vi "Generate Tree Data Representation.vi"(8 "error in (no error)":errorcluster, 11 "ParseGDSII in":refnum<class "ParseGDSII.lvclass">) -> (0 "error out":errorcluster, 3 "ParseGDSII out":refnum<class "ParseGDSII.lvclass">)   [LabVIEW 2019, in "ParseGDSII.lvclass"]
uses:
  ParseGDSII.lvclass
  Tree/Tree.lvclass
  ParseGDSII.lvclass/ParseGDSII.ctl
  Fast Tree/Fast Tree.lvclass
  DataTypes/Base/GDSII.DataType.lvclass
panel:
  out "sum 3":u32
  out "sum 2":u32
  out "sum":u32
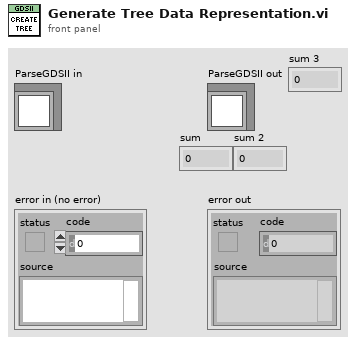
[diagram p1: front panel]
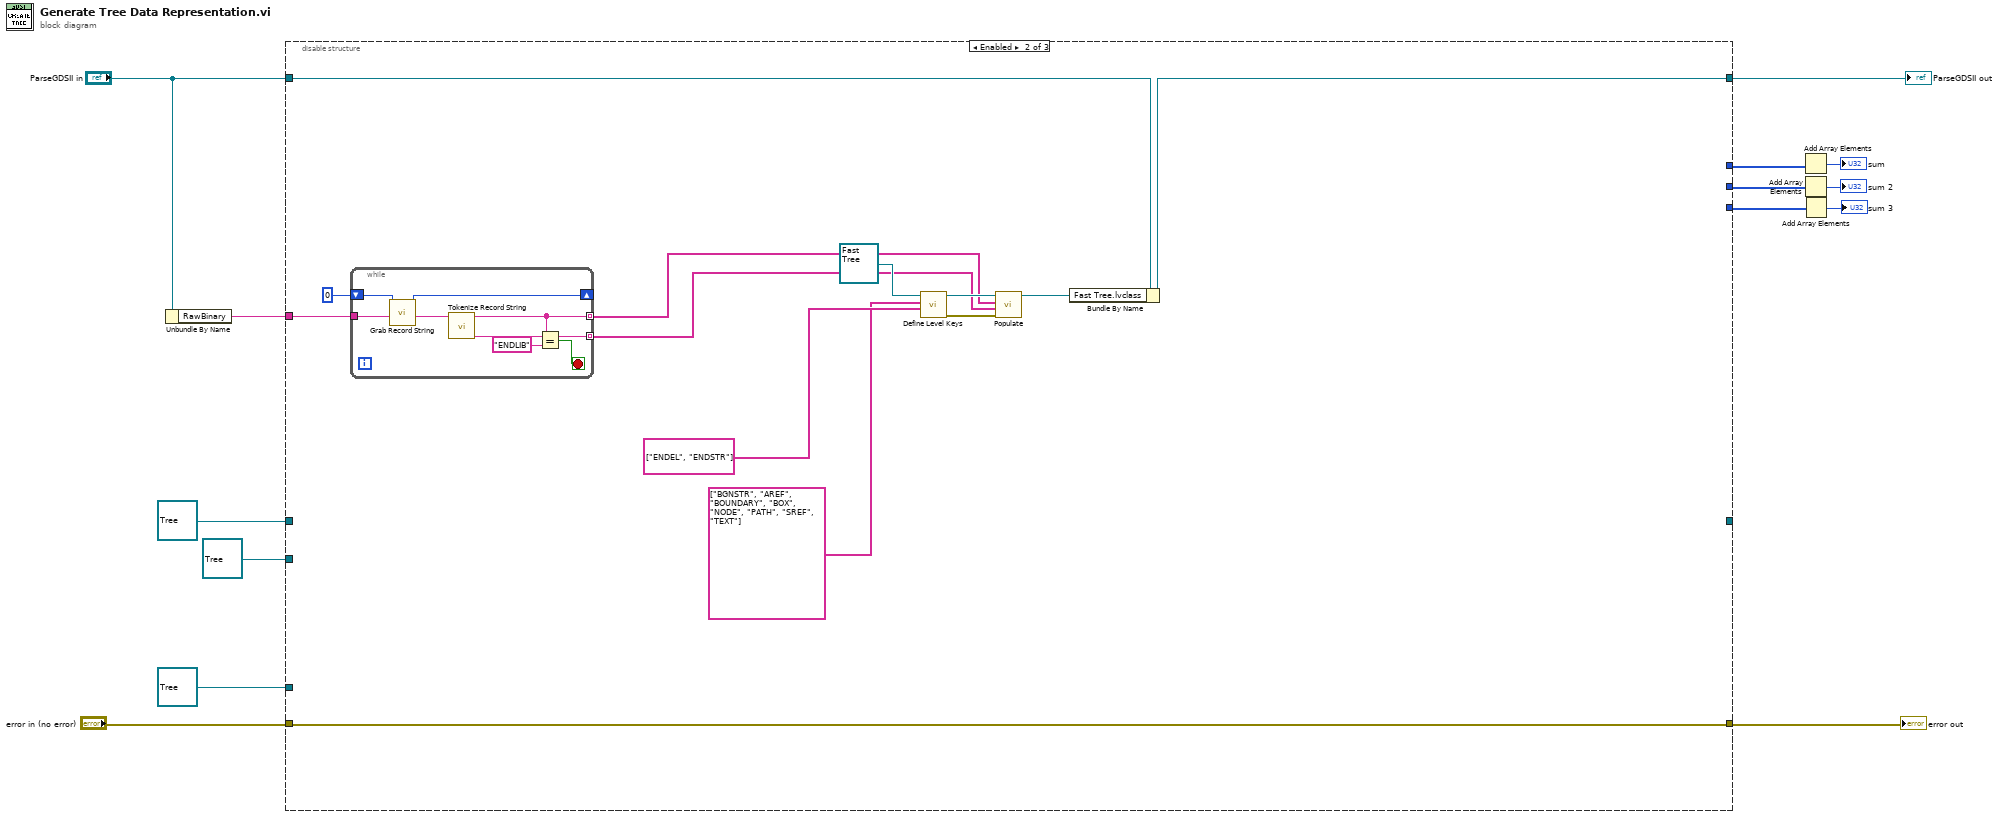
[diagram p0: block diagram]
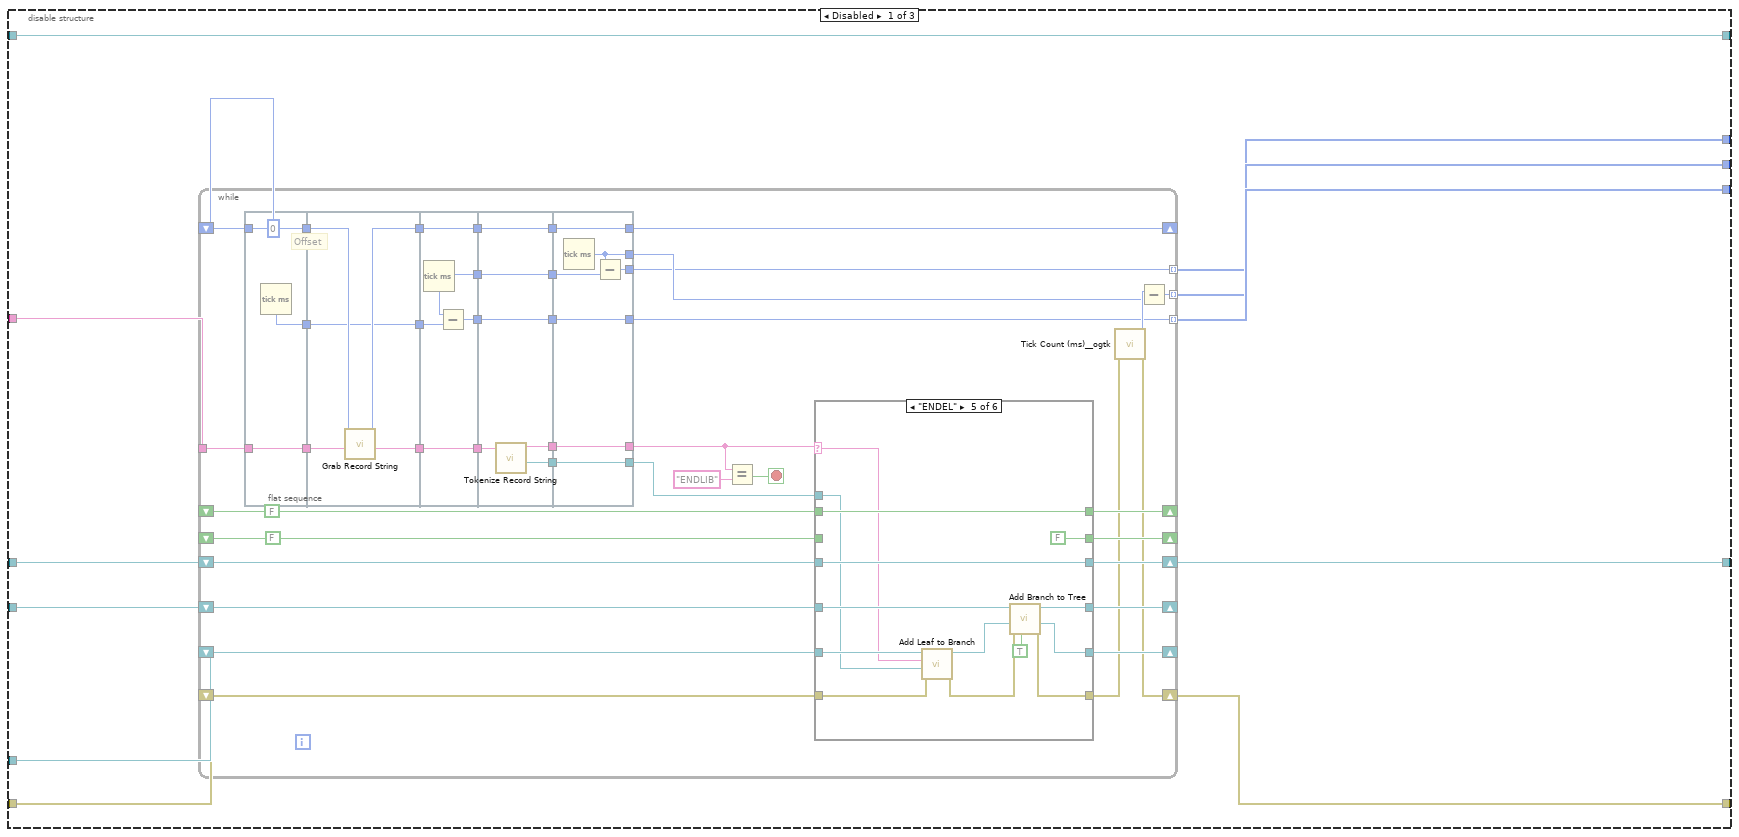
[diagram p2: hidden frame]
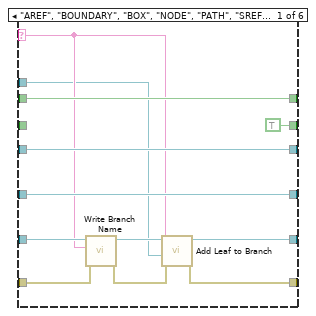
[diagram p3: hidden frame]
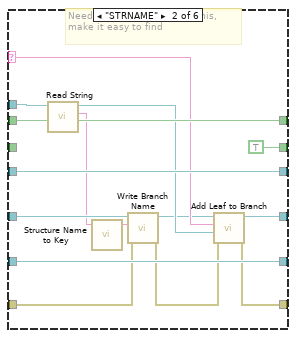
[diagram p4: hidden frame]
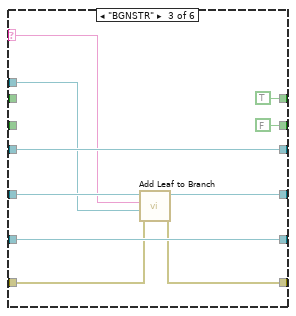
[diagram p5: hidden frame]
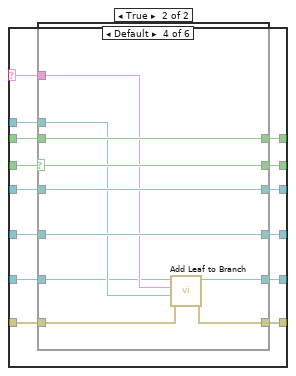
[diagram p6: hidden frame]
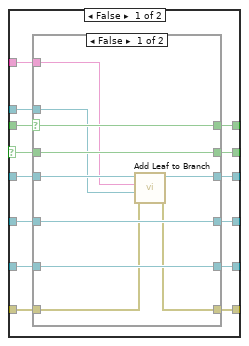
[diagram p7: hidden frame]
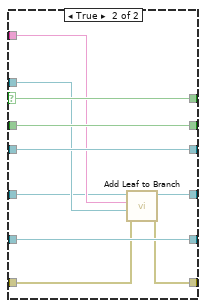
[diagram p8: hidden frame]
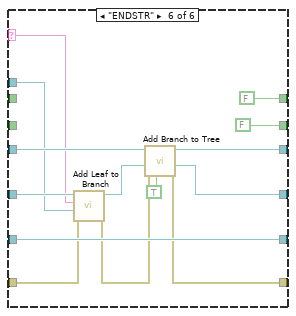
[diagram p9: hidden frame]
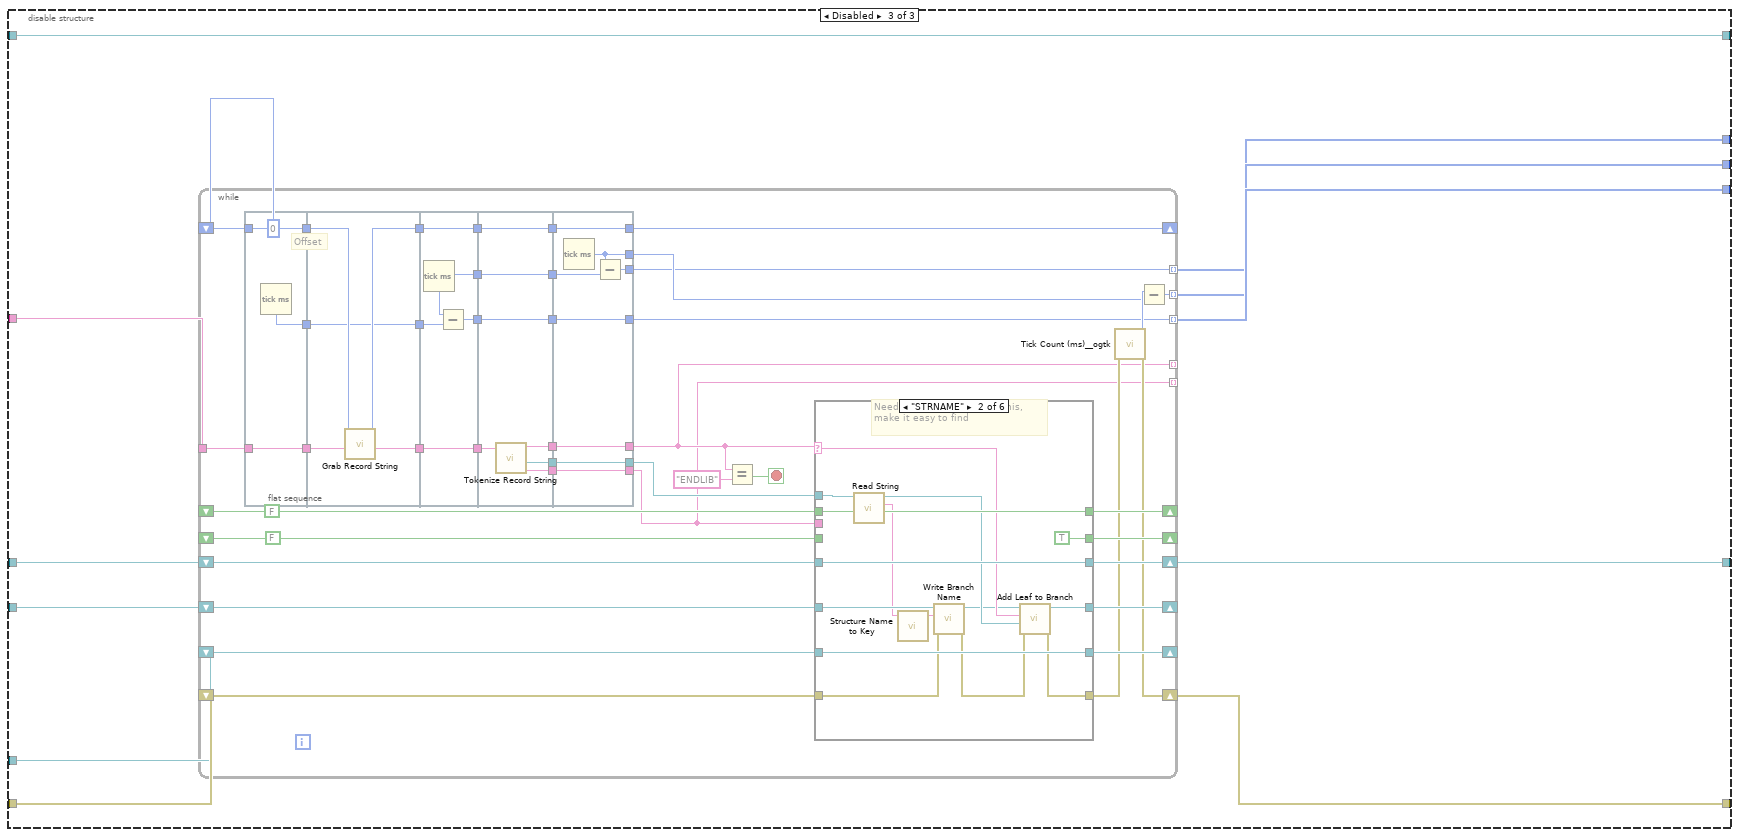
[diagram p10: hidden frame]
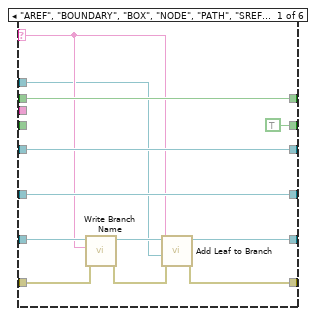
[diagram p11: hidden frame]
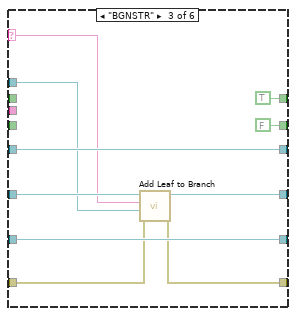
[diagram p12: hidden frame]
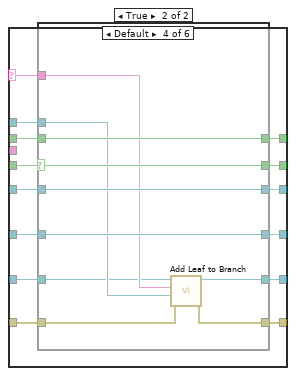
[diagram p13: hidden frame]
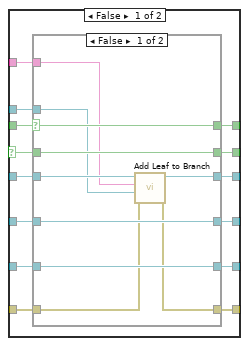
[diagram p14: hidden frame]
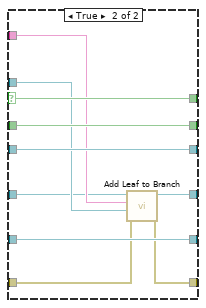
[diagram p15: hidden frame]
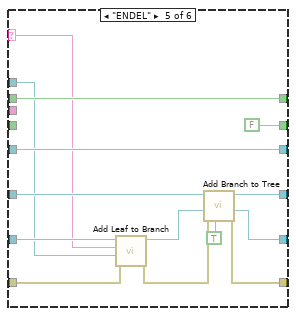
[diagram p16: hidden frame]
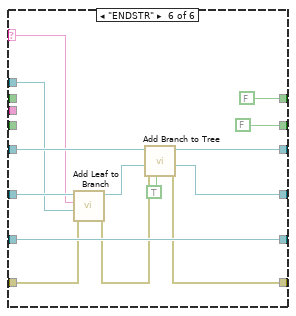
[diagram p17: hidden frame]
diagram:
  n1 = Unbundle By Name("ParseGDSII in") -> ("RawBinary"=w11:string)
  n2 = disable-structure shown="Enabled" {
    disable-tunnel: refnum<class "Tree.lvclass"> refnum ("Root out") -> [w26 _ w242]
    disable-tunnel: refnum<class "Tree.lvclass"> refnum ("Branch out") -> [w25 _ w241]
    disable-tunnel: refnum<class "Tree.lvclass"> refnum ("Branch out") -> [w24 _ w240]
    disable-tunnel: w11 -> [w23 w225 w250]
    disable-tunnel: [w21 _ w248] -> _
    disable-tunnel: [w20 w230 w247] -> w10
    disable-tunnel: "error in (no error)" -> [w19 w230 w246]
    disable-tunnel: [w18 _ w245] -> w8
    disable-tunnel: [w17 _ w244] -> w7
    disable-tunnel: [w16 _ w243] -> w6
    disable-tunnel: "ParseGDSII in" -> [w15 w220 w239]
    disable-tunnel: [w15 w218 w239] -> w1
    frame Disabled {
      n3 = while {
        tunnel: w23 -> [w57]
        shift-right: [w54] -> _
        shift-left: 0 ("New Offset") -> [w53]
        shift-right: [w64] -> _
        shift-left: FALSE -> [w65]
        shift-right: [w66] -> _
        shift-left: FALSE -> [w67]
        shift-right: [w59] -> w21
        shift-left: w26 -> [w60]
        shift-right: [w61] -> _
        shift-left: w25 -> [w62]
        shift-right: [w63] -> _
        shift-left: w24 -> [w68]
        shift-right: [w40] -> w20
        shift-left: w19 -> [w55]
        tunnel: [w33] -> w17 mode=indexing
        tunnel: [w32] -> w16 mode=indexing
        tunnel: [w31] -> w18 mode=indexing
        stop <- w56 stop-if-true
        n4 = flat-sequence {
          tunnel: w53 -> [w70]
          tunnel: w57 -> [w71]
          tunnel: [w71] -> w52
          tunnel: [w70] -> w51
          tunnel: [w69] -> w37
          tunnel: w52 -> [w75]
          tunnel: w51 -> [w73]
          tunnel: [w76] -> w45
          tunnel: [w74] -> w43
          tunnel: w37 -> [w72]
          tunnel: [w72] -> w36
          tunnel: w45 -> [w81]
          tunnel: [w81] -> w44
          tunnel: w43 -> [w80]
          tunnel: [w80] -> w42
          tunnel: [w79] -> w39
          tunnel: w36 -> [w78]
          tunnel: [w77] -> w29
          tunnel: w44 -> [w86]
          tunnel: w42 -> [w87]
          tunnel: [w87] -> w48
          tunnel: [w85] -> w47
          tunnel: [w84] -> w46
          tunnel: w39 -> [w83]
          tunnel: [w83] -> w38
          tunnel: [w82] -> w30
          tunnel: w29 -> [w82]
          tunnel: [w92] -> w49
          tunnel: [w93] -> w50
          tunnel: [w94] -> w54
          tunnel: w48 -> [w94]
          tunnel: w47 -> [w93]
          tunnel: w46 -> [w92]
          tunnel: w38 -> [w91]
          tunnel: [w90] -> w34
          tunnel: [w89] -> w32
          tunnel: [w88] -> w31
          tunnel: w30 -> [w88]
          frame #0 {
            n5 = Tick Count (ms)() -> (millisecond timer value=w69:u32)
          }
          frame #1 {
            # "Offset"
            n6 = call "Grab Record String.vi"("Raw Binary String"=w75, "Offset"=w73) -> ("Record String"=w76:string, "New Offset"=w74:i32)  [unwired: 8 in]
          }
          frame #2 {
            n7 = Tick Count (ms)() -> (millisecond timer value=w79:u32)
            n8 = Subtract(x=w79, y=w78) -> (x-y=w77:u32)
          }
          frame #3 {
            n9 = call "Tokenize Record String.vi"("Record String"=w86) -> ("Payload"=w85:refnum<class "GDSII.DataType.lvclass">, "Record Type"=w84:string)  [unwired: 7 in, 2 out]
          }
          frame #4 {
            n10 = Tick Count (ms)() -> (millisecond timer value=w90:u32)
            n11 = Subtract(x=w90, y=w91) -> (x-y=w89:u32)
          }
        }
        n12 = Equal?(x=w49, y="ENDLIB") -> (x = y?=w56:bool)
        n13 = case shown="\"ENDEL\"" w49 {
          selector: w49 -> [w99 w115 w125 w134 w194 w208]
          tunnel: w67 -> [_ _ _ w142 _ _]
          tunnel: [TRUE TRUE FALSE w141 FALSE FALSE] -> w66
          tunnel: w50 -> [w98 w118 w124 w143 w195 w210]
          tunnel: [w100 w117 w128 w144 w199 w215] -> w63
          tunnel: w68 -> [w102 w117 w128 w145 w196 w215]
          tunnel: w65 -> [w105 w120 _ w140 w202 _]
          tunnel: [w105 w120 TRUE w139 w202 FALSE] -> w64
          tunnel: w62 -> [w104 w113 w126 w138 w198 w211]
          tunnel: [w104 w116 w127 w137 w200 w212] -> w61
          tunnel: [w103 w119 w130 w135 w201 w214] -> w59
          tunnel: w60 -> [w103 w119 w130 w136 w201 w213]
          tunnel: w55 -> [w95 w109 w123 w133 w191 w207]
          tunnel: [w96 w107 w122 w132 w193 w205] -> w41
          frame "AREF", "BOUNDARY", "BOX", "NODE", "PATH", "SREF", "TEXT" {
            n14 = call "Write Branch Name.vi"("error in"=w95, "Name"=w99, "Tree in"=w102) -> ("error out"=w97:errorcluster, "Tree out"=w101:refnum<class "Tree.lvclass">)  [unwired: 7 in]
            n15 = call "Add Leaf to Branch.vi"("error in"=w97, "Item"=w98, "Name"=w99, "Tree in"=w101) -> ("error out"=w96:errorcluster, "Tree out"=w100:refnum<class "Tree.lvclass">)  [unwired: 6 in]
          }
          frame "STRNAME" {
            # "Need to reference back to this, make it easy to find"
            n16 = call-dynamic "Read String.vi"("GDSII.DataType in"=w118) -> ("String"=w110:string, "GDSII.DataType out"=w114:refnum<class "GDSII.DataType.lvclass">)  [unwired: 9 in]
            n17 = call "Structure Name to Key.vi"("Name"=w110) -> ("Key"=w111:string)  [unwired: 4 in]
            n18 = call "Write Branch Name.vi"("error in"=w109, "Name"=w111, "Tree in"=w113) -> ("error out"=w108:errorcluster, "Tree out"=w112:refnum<class "Tree.lvclass">)  [unwired: 7 in]
            n19 = call "Add Leaf to Branch.vi"("error in"=w108, "Item"=w114, "Name"=w115, "Tree in"=w112) -> ("error out"=w107:errorcluster, "Tree out"=w116:refnum<class "Tree.lvclass">)  [unwired: 6 in]
          }
          frame "BGNSTR" {
            n20 = call "Add Leaf to Branch.vi"("error in"=w123, "Item"=w124, "Name"=w125, "Tree in"=w126) -> ("error out"=w122:errorcluster, "Tree out"=w127:refnum<class "Tree.lvclass">)  [unwired: 6 in]
          }
          frame Default {
            n21 = case shown="True" w142 {
              selector: w142 -> [w156 w189]
              tunnel: w145 -> [w154 w182]
              tunnel: [w155 w185] -> w144
              tunnel: w143 -> [w151 w184]
              tunnel: [w157 w189] -> w141
              tunnel: w140 -> [w159 w186]
              tunnel: [w158 w186] -> w139
              tunnel: w138 -> [w153 w187]
              tunnel: [w152 w187] -> w137
              tunnel: w136 -> [w150 w188]
              tunnel: [w149 w188] -> w135
              tunnel: w134 -> [w148 w183]
              tunnel: w133 -> [w147 w181]
              tunnel: [w146 w180] -> w132
              frame False {
                n22 = case shown="False" w159 {
                  selector: w159 -> [w168 w179]
                  tunnel: [w168 w179] -> w158
                  tunnel: [w167 w178] -> w157
                  tunnel: w156 -> [w167 w178]
                  tunnel: [w166 w177] -> w155
                  tunnel: w154 -> [w166 w177]
                  tunnel: w153 -> [w169 w172]
                  tunnel: [w169 w175] -> w152
                  tunnel: w151 -> [w163 w173]
                  tunnel: w150 -> [w165 w176]
                  tunnel: [w164 w176] -> w149
                  tunnel: w148 -> [w162 w174]
                  tunnel: w147 -> [w161 w171]
                  tunnel: [w160 w170] -> w146
                  frame False {
                    n23 = call "Add Leaf to Branch.vi"("error in"=w161, "Item"=w163, "Name"=w162, "Tree in"=w165) -> ("error out"=w160:errorcluster, "Tree out"=w164:refnum<class "Tree.lvclass">)  [unwired: 6 in]
                  }
                  frame True {
                    n24 = call "Add Leaf to Branch.vi"("error in"=w171, "Item"=w173, "Name"=w174, "Tree in"=w172) -> ("error out"=w170:errorcluster, "Tree out"=w175:refnum<class "Tree.lvclass">)  [unwired: 6 in]
                  }
                }
              }
              frame True {
                n25 = call "Add Leaf to Branch.vi"("error in"=w181, "Item"=w184, "Name"=w183, "Tree in"=w182) -> ("error out"=w180:errorcluster, "Tree out"=w185:refnum<class "Tree.lvclass">)  [unwired: 6 in]
              }
            }
          }
          frame "ENDEL" {
            n26 = call "Add Leaf to Branch.vi"("error in"=w191, "Item"=w195, "Name"=w194, "Tree in"=w196) -> ("error out"=w192:errorcluster, "Tree out"=w197:refnum<class "Tree.lvclass">)  [unwired: 6 in]
            n27 = call "Add Branch to Tree.vi"("Truncate Branch?"=TRUE, "error in"=w192, "Branch in"=w197, "Root in"=w198) -> ("error out"=w193:errorcluster, "Branch out"=w199:refnum<class "Tree.lvclass">, "Root out"=w200:refnum<class "Tree.lvclass">)  [unwired: 5 in]
          }
          frame "ENDSTR" {
            n28 = call "Add Leaf to Branch.vi"("error in"=w207, "Item"=w210, "Name"=w208, "Tree in"=w211) -> ("error out"=w206:errorcluster, "Tree out"=w209:refnum<class "Tree.lvclass">)  [unwired: 6 in]
            n29 = call "Add Branch to Tree.vi"("Truncate Branch?"=TRUE, "error in"=w206, "Branch in"=w209, "Root in"=w213) -> ("error out"=w205:errorcluster, "Branch out"=w212:refnum<class "Tree.lvclass">, "Root out"=w214:refnum<class "Tree.lvclass">)  [unwired: 5 in]
          }
        }
        n30 = call <userlib>:"Tick Count (ms)__ogtk.vi"("error in (no error)"=w41) -> ("error out"=w40:errorcluster, "millisecond timer value"=w35:u32)  [unwired: 9 in]
        n31 = Subtract(x=w35, y=w34) -> (x-y=w33:u32)
      }
    }
    frame Enabled {
      n32 = while {
        tunnel: [w235] -> w224 mode=indexing
        tunnel: [w234] -> w223 mode=indexing
        shift-right: [w232] -> _
        shift-left: 0 ("New Offset") -> [w233]
        tunnel: w225 -> [w231]
        stop <- w236 stop-if-true
        n33 = call "Grab Record String.vi"("Raw Binary String"=w231, "Offset"=w233) -> ("Record String"=w237:string, "New Offset"=w232:i32)  [unwired: 8 in]
        n34 = call "Tokenize Record String.vi"("Record String"=w237) -> ("Payload Binary"=w234:string, "Record Type"=w235:string)  [unwired: 7 in, 2 out]
        n35 = Equal?(x=w235, y="ENDLIB") -> (x = y?=w236:bool)
      }
      n36 = call "Define Level Keys.vi"("Level Down Keys"=string[] ["ENDEL", "ENDSTR"], "Level Up Keys"=string[] ["BGNSTR", "AREF", "BOUNDARY", "BOX", "NODE", "PATH", "SREF", "TEXT"], "Fast Tree in"=refnum<class "Fast Tree.lvclass"> refnum) -> ("error out"=w228:errorcluster, "Fast Tree out"=w229:refnum<class "Fast Tree.lvclass">)  [unwired: 7 in]
      n37 = call "Populate.vi"("error in"=w228, "Values In"=w223, "Keys In"=w224, "Fast Tree in"=w229) -> ("Fast Tree out"=w219:refnum<class "Fast Tree.lvclass">)  [unwired: 5 in, 2 out]
      n38 = Bundle By Name(cluster=w220, "Fast Tree.lvclass"=w219) -> (w218:refnum<class "ParseGDSII.lvclass">)
    }
    frame Disabled {
      n39 = while {
        tunnel: w250 -> [w283]
        shift-right: [w280] -> _
        shift-left: 0 ("New Offset") -> [w279]
        shift-right: [w290] -> _
        shift-left: FALSE -> [w291]
        shift-right: [w292] -> _
        shift-left: FALSE -> [w293]
        shift-right: [w285] -> w248
        shift-left: w242 -> [w286]
        shift-right: [w287] -> _
        shift-left: w241 -> [w288]
        shift-right: [w289] -> _
        shift-left: w240 -> [w294]
        shift-right: [w267] -> w247
        shift-left: w246 -> [w281]
        tunnel: [w260] -> w244 mode=indexing
        tunnel: [w259] -> w243 mode=indexing
        tunnel: [w258] -> w245 mode=indexing
        tunnel: [w254] -> _ mode=indexing
        tunnel: [w253] -> _ mode=indexing
        stop <- w282 stop-if-true
        n40 = flat-sequence {
          tunnel: w279 -> [w296]
          tunnel: w283 -> [w297]
          tunnel: [w297] -> w278
          tunnel: [w296] -> w277
          tunnel: [w295] -> w264
          tunnel: w278 -> [w301]
          tunnel: w277 -> [w299]
          tunnel: [w302] -> w272
          tunnel: [w300] -> w270
          tunnel: w264 -> [w298]
          tunnel: [w298] -> w263
          tunnel: w272 -> [w307]
          tunnel: [w307] -> w271
          tunnel: w270 -> [w306]
          tunnel: [w306] -> w269
          tunnel: [w305] -> w266
          tunnel: w263 -> [w304]
          tunnel: [w303] -> w256
          tunnel: w271 -> [w313]
          tunnel: w269 -> [w314]
          tunnel: [w314] -> w275
          tunnel: [w312] -> w274
          tunnel: [w311] -> w273
          tunnel: w266 -> [w310]
          tunnel: [w310] -> w265
          tunnel: [w309] -> w257
          tunnel: w256 -> [w309]
          tunnel: [w308] -> w255
          tunnel: [w320] -> w254
          tunnel: [w321] -> w276
          tunnel: [w322] -> w280
          tunnel: w275 -> [w322]
          tunnel: w274 -> [w321]
          tunnel: w273 -> [w320]
          tunnel: w265 -> [w319]
          tunnel: [w318] -> w261
          tunnel: [w317] -> w259
          tunnel: [w316] -> w258
          tunnel: w257 -> [w316]
          tunnel: [w315] -> w253
          tunnel: w255 -> [w315]
          frame #0 {
            n41 = Tick Count (ms)() -> (millisecond timer value=w295:u32)
          }
          frame #1 {
            # "Offset"
            n42 = call "Grab Record String.vi"("Raw Binary String"=w301, "Offset"=w299) -> ("Record String"=w302:string, "New Offset"=w300:i32)  [unwired: 8 in]
          }
          frame #2 {
            n43 = Tick Count (ms)() -> (millisecond timer value=w305:u32)
            n44 = Subtract(x=w305, y=w304) -> (x-y=w303:u32)
          }
          frame #3 {
            n45 = call "Tokenize Record String.vi"("Record String"=w313) -> ("Payload Binary"=w308:string, "Payload"=w312:refnum<class "GDSII.DataType.lvclass">, "Record Type"=w311:string)  [unwired: 7 in, 1 out]
          }
          frame #4 {
            n46 = Tick Count (ms)() -> (millisecond timer value=w318:u32)
            n47 = Subtract(x=w318, y=w319) -> (x-y=w317:u32)
          }
        }
        n48 = Equal?(x=w254, y="ENDLIB") -> (x = y?=w282:bool)
        n49 = case shown="\"STRNAME\"" w254 {
          selector: w254 -> [w327 w343 w353 w362 w422 w436]
          tunnel: w293 -> [_ _ _ w370 _ _]
          tunnel: [TRUE TRUE FALSE w369 FALSE FALSE] -> w292
          tunnel: w276 -> [w326 w346 w352 w371 w423 w438]
          tunnel: [w328 w345 w356 w372 w427 w443] -> w289
          tunnel: w294 -> [w330 w345 w356 w373 w424 w443]
          tunnel: w291 -> [w333 w348 _ w368 w430 _]
          tunnel: [w333 w348 TRUE w367 w430 FALSE] -> w290
          tunnel: w288 -> [w332 w341 w354 w366 w426 w439]
          tunnel: [w332 w344 w355 w365 w428 w440] -> w287
          tunnel: [w331 w347 w358 w363 w429 w442] -> w285
          tunnel: w286 -> [w331 w347 w358 w364 w429 w441]
          tunnel: w281 -> [w323 w337 w351 w361 w419 w435]
          tunnel: [w324 w335 w350 w360 w421 w433] -> w268
          tunnel: w253 -> [_ _ _ _ _ _]
          frame "AREF", "BOUNDARY", "BOX", "NODE", "PATH", "SREF", "TEXT" {
            n50 = call "Write Branch Name.vi"("error in"=w323, "Name"=w327, "Tree in"=w330) -> ("error out"=w325:errorcluster, "Tree out"=w329:refnum<class "Tree.lvclass">)  [unwired: 7 in]
            n51 = call "Add Leaf to Branch.vi"("error in"=w325, "Item"=w326, "Name"=w327, "Tree in"=w329) -> ("error out"=w324:errorcluster, "Tree out"=w328:refnum<class "Tree.lvclass">)  [unwired: 6 in]
          }
          frame "STRNAME" {
            # "Need to reference back to this, make it easy to find"
            n52 = call-dynamic "Read String.vi"("GDSII.DataType in"=w346) -> ("String"=w338:string, "GDSII.DataType out"=w342:refnum<class "GDSII.DataType.lvclass">)  [unwired: 9 in]
            n53 = call "Structure Name to Key.vi"("Name"=w338) -> ("Key"=w339:string)  [unwired: 4 in]
            n54 = call "Write Branch Name.vi"("error in"=w337, "Name"=w339, "Tree in"=w341) -> ("error out"=w336:errorcluster, "Tree out"=w340:refnum<class "Tree.lvclass">)  [unwired: 7 in]
            n55 = call "Add Leaf to Branch.vi"("error in"=w336, "Item"=w342, "Name"=w343, "Tree in"=w340) -> ("error out"=w335:errorcluster, "Tree out"=w344:refnum<class "Tree.lvclass">)  [unwired: 6 in]
          }
          frame "BGNSTR" {
            n56 = call "Add Leaf to Branch.vi"("error in"=w351, "Item"=w352, "Name"=w353, "Tree in"=w354) -> ("error out"=w350:errorcluster, "Tree out"=w355:refnum<class "Tree.lvclass">)  [unwired: 6 in]
          }
          frame Default {
            n57 = case shown="True" w370 {
              selector: w370 -> [w384 w417]
              tunnel: w373 -> [w382 w410]
              tunnel: [w383 w413] -> w372
              tunnel: w371 -> [w379 w412]
              tunnel: [w385 w417] -> w369
              tunnel: w368 -> [w387 w414]
              tunnel: [w386 w414] -> w367
              tunnel: w366 -> [w381 w415]
              tunnel: [w380 w415] -> w365
              tunnel: w364 -> [w378 w416]
              tunnel: [w377 w416] -> w363
              tunnel: w362 -> [w376 w411]
              tunnel: w361 -> [w375 w409]
              tunnel: [w374 w408] -> w360
              frame False {
                n58 = case shown="False" w387 {
                  selector: w387 -> [w396 w407]
                  tunnel: [w396 w407] -> w386
                  tunnel: [w395 w406] -> w385
                  tunnel: w384 -> [w395 w406]
                  tunnel: [w394 w405] -> w383
                  tunnel: w382 -> [w394 w405]
                  tunnel: w381 -> [w397 w400]
                  tunnel: [w397 w403] -> w380
                  tunnel: w379 -> [w391 w401]
                  tunnel: w378 -> [w393 w404]
                  tunnel: [w392 w404] -> w377
                  tunnel: w376 -> [w390 w402]
                  tunnel: w375 -> [w389 w399]
                  tunnel: [w388 w398] -> w374
                  frame False {
                    n59 = call "Add Leaf to Branch.vi"("error in"=w389, "Item"=w391, "Name"=w390, "Tree in"=w393) -> ("error out"=w388:errorcluster, "Tree out"=w392:refnum<class "Tree.lvclass">)  [unwired: 6 in]
                  }
                  frame True {
                    n60 = call "Add Leaf to Branch.vi"("error in"=w399, "Item"=w401, "Name"=w402, "Tree in"=w400) -> ("error out"=w398:errorcluster, "Tree out"=w403:refnum<class "Tree.lvclass">)  [unwired: 6 in]
                  }
                }
              }
              frame True {
                n61 = call "Add Leaf to Branch.vi"("error in"=w409, "Item"=w412, "Name"=w411, "Tree in"=w410) -> ("error out"=w408:errorcluster, "Tree out"=w413:refnum<class "Tree.lvclass">)  [unwired: 6 in]
              }
            }
          }
          frame "ENDEL" {
            n62 = call "Add Leaf to Branch.vi"("error in"=w419, "Item"=w423, "Name"=w422, "Tree in"=w424) -> ("error out"=w420:errorcluster, "Tree out"=w425:refnum<class "Tree.lvclass">)  [unwired: 6 in]
            n63 = call "Add Branch to Tree.vi"("Truncate Branch?"=TRUE, "error in"=w420, "Branch in"=w425, "Root in"=w426) -> ("error out"=w421:errorcluster, "Branch out"=w427:refnum<class "Tree.lvclass">, "Root out"=w428:refnum<class "Tree.lvclass">)  [unwired: 5 in]
          }
          frame "ENDSTR" {
            n64 = call "Add Leaf to Branch.vi"("error in"=w435, "Item"=w438, "Name"=w436, "Tree in"=w439) -> ("error out"=w434:errorcluster, "Tree out"=w437:refnum<class "Tree.lvclass">)  [unwired: 6 in]
            n65 = call "Add Branch to Tree.vi"("Truncate Branch?"=TRUE, "error in"=w434, "Branch in"=w437, "Root in"=w441) -> ("error out"=w433:errorcluster, "Branch out"=w440:refnum<class "Tree.lvclass">, "Root out"=w442:refnum<class "Tree.lvclass">)  [unwired: 5 in]
          }
        }
        n66 = call <userlib>:"Tick Count (ms)__ogtk.vi"("error in (no error)"=w268) -> ("error out"=w267:errorcluster, "millisecond timer value"=w262:u32)  [unwired: 9 in]
        n67 = Subtract(x=w262, y=w261) -> (x-y=w260:u32)
      }
    }
  }
  "error out" <- w10
  "ParseGDSII out" <- w1
  n68 = Add Array Elements(numeric array=w6) -> (sum=→"sum":u32)
  n69 = Add Array Elements(numeric array=w7) -> (sum=→"sum 2":u32)
  n70 = Add Array Elements(numeric array=w8) -> (sum=→"sum 3":u32)
